vi "Decode.vi"(8 "error in (no error)":errorcluster, 10 "Clear Raw Data":bool caption="Clear Raw Data(False)", 11 "Raw Data":string) -> (0 "error out":errorcluster, 1 "Success":bool, 2 "Sequence No":string, 3 "Data":string)   [LabVIEW 2019, in "GaitDAQ UI.lvlib"]
uses:
  GaitDAQ UI.lvlib
  Step.ctl
  Sign.ctl
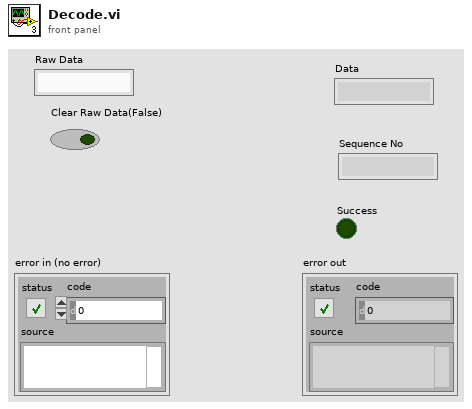
[diagram p1: front panel]
types:
  T1 = typedef "GaitDAQ UI.lvlib/Step.ctl" = enum16{"找A帧头", "找A序号", "找A数据", "找B帧头", "找B序号", "找B数据"}
  T2 = typedef "GaitDAQ UI.lvlib/Sign.ctl" = i32
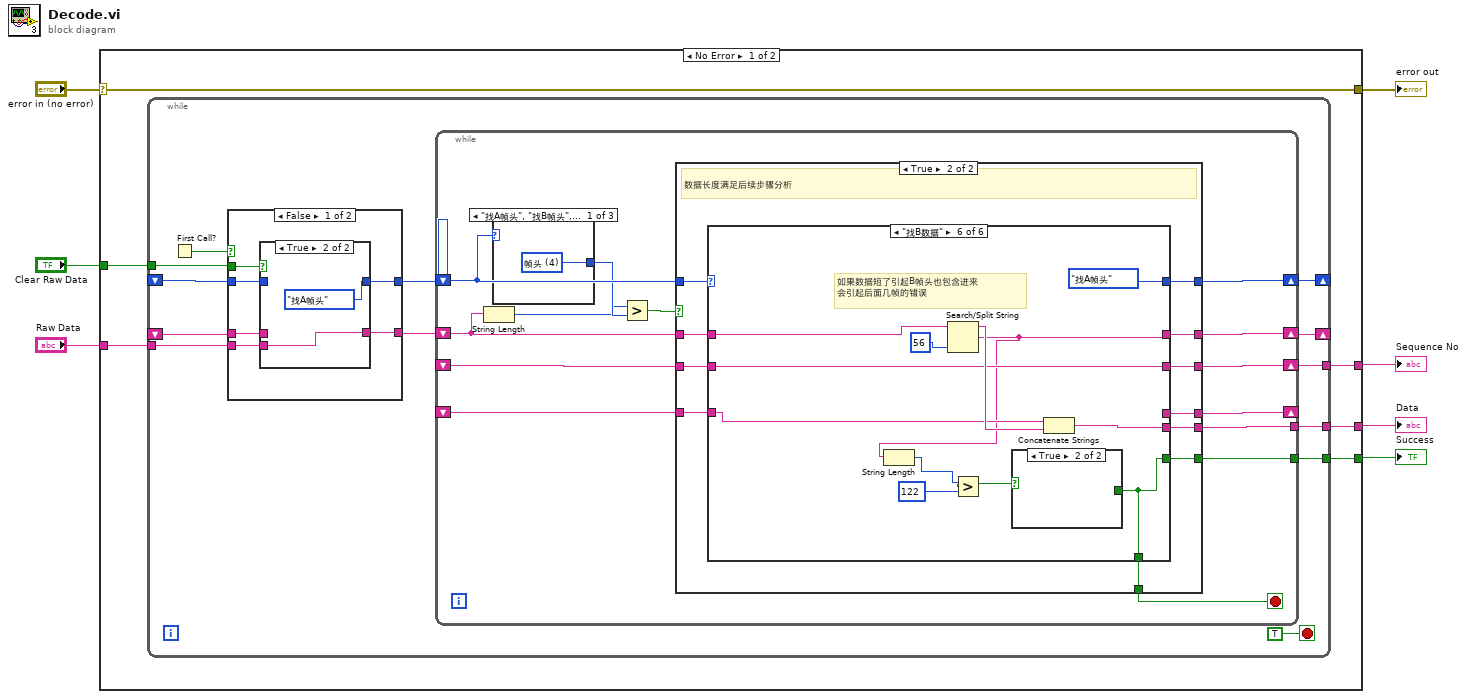
[diagram p0: block diagram]
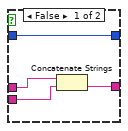
[diagram p2: hidden frame]
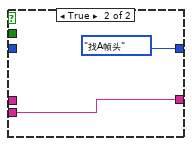
[diagram p3: hidden frame]
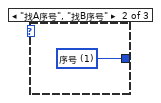
[diagram p4: hidden frame]
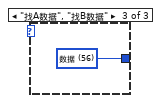
[diagram p5: hidden frame]
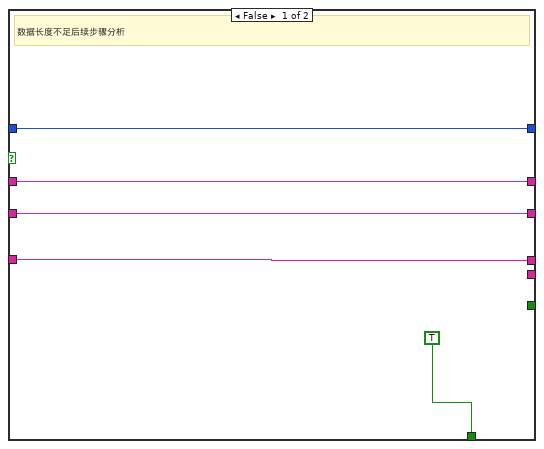
[diagram p6: hidden frame]
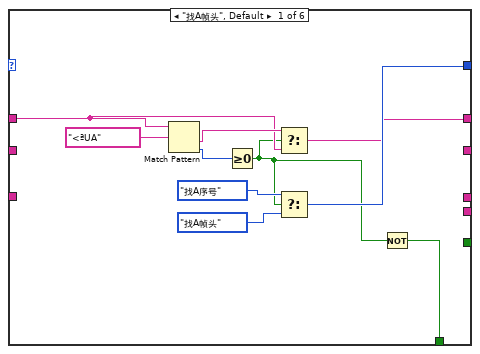
[diagram p7: hidden frame]
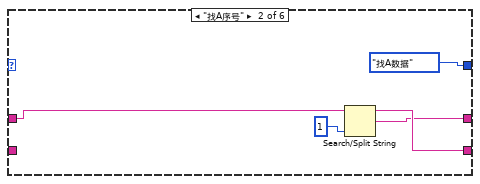
[diagram p8: hidden frame]
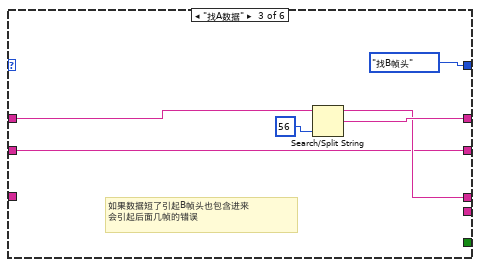
[diagram p9: hidden frame]
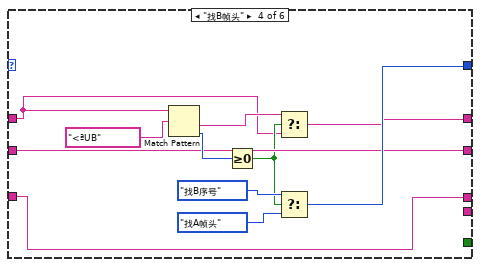
[diagram p10: hidden frame]
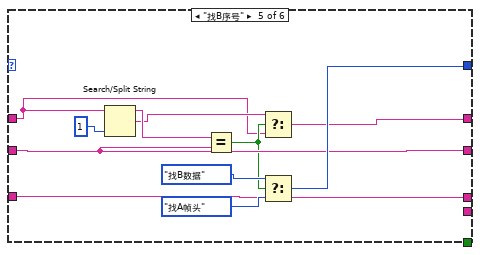
[diagram p11: hidden frame]
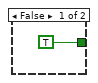
[diagram p12: hidden frame]
diagram:
  n1 = case shown="No Error" "error in (no error)" {
    selector: "error in (no error)" -> [w8 w130]
    tunnel: "Raw Data" -> [w13 _]
    tunnel: "Clear Raw Data" -> [w12 _]
    tunnel: [w11 _] -> w5
    tunnel: [w10 _] -> w4
    tunnel: [w9 _] -> w3
    tunnel: [w8 w130] -> w1
    frame No Error {
      n2 = while {
        tunnel: [w25] -> w9
        shift-right: [w26] -> _
        shift-left: _ -> [w15]
        tunnel: [w24] -> w10
        tunnel: [w23] -> w11
        tunnel: w13 -> [w16]
        tunnel: w12 -> [w17]
        shift-right: [w18] -> _
        shift-left: _ -> [w19]
        stop <- TRUE stop-if-true
        n3 = First Call?() -> (First Call?: T/F=w21:bool)
        n4 = case shown="False" w21 {
          tunnel: [w27 Step."找A帧头"] -> w20
          tunnel: w19 -> [w28 _]
          tunnel: w17 -> [w32 _]
          tunnel: w16 -> [w31 w39]
          tunnel: w15 -> [w30 _]
          tunnel: [w29 w39] -> w14
          frame False {
            n5 = case shown="True" w32 {
              tunnel: [w36 w38] -> w29
              tunnel: w31 -> [w35 w38]
              tunnel: w30 -> [w34 _]
              tunnel: w28 -> [w33 _]
              tunnel: [w33 Step."找A帧头"] -> w27
              frame False {
                n6 = Concatenate Strings(w34, w35) -> (w36:string)
              }
              frame True {
              }
            }
          }
          frame True {
          }
        }
        n7 = while {
          shift-right: [w53] -> w18
          shift-left: w20 -> [w51]
          shift-right: [w52] -> w26
          shift-left: w14 -> [w54]
          shift-right: [w46] -> w25
          shift-left: _ -> [w45]
          shift-right: [w44] -> _
          shift-left: _ -> [w43]
          tunnel: [w42] -> w23
          tunnel: [w41] -> w24
          stop <- w47 stop-if-true
          n8 = String Length(string=w54) -> (length=w49:i32)
          n9 = case shown="\"找A帧头\", \"找B帧头\", Default" w51 {
            tunnel: [w55 w56 w57] -> w50
            frame "找A帧头", "找B帧头", Default {
              w55 = T2 4 items=["帧头"=4, "序号"=1, "数据"=56]
            }
            frame "找A序号", "找B序号" {
              w56 = T2 1 items=["帧头"=4, "序号"=1, "数据"=56]
            }
            frame "找A数据", "找B数据" {
              w57 = T2 56 items=["帧头"=4, "序号"=1, "数据"=56]
            }
          }
          n10 = Greater?(x=w49, y=w50) -> (0:w48:bool)
          n11 = case shown="True" w48 {
            tunnel: w51 -> [w61 w73]
            tunnel: w54 -> [w62 w72]
            tunnel: [w61 w71] -> w53
            tunnel: [w62 w70] -> w52
            tunnel: [TRUE w67] -> w47
            tunnel: [w59 w69] -> w46
            tunnel: w45 -> [w59 w68]
            tunnel: [w58 w66] -> w44
            tunnel: w43 -> [w58 w65]
            tunnel: [_ w64] -> w42
            tunnel: [_ w63] -> w41
            frame False {
              # "数据长度不足后续步骤分析"
            }
            frame True {
              # "数据长度满足后续步骤分析"
              n12 = case shown="\"找B数据\"" w73 {
                tunnel: w72 -> [w76 w87 w90 w96 w108 w127]
                tunnel: [w80 Step."找A数据" Step."找B帧头" ("f") w102 w113 Step."找A帧头" ("f")] -> w71
                tunnel: [w78 w85 w93 w97 w107 w121] -> w70
                tunnel: [_ w86 w89 w101 w112 w122] -> w69
                tunnel: w68 -> [_ _ w89 w101 w112 w122]
                tunnel: [w75 _ _ _ _ w117] -> w67
                tunnel: [_ _ w92 w95 w106 _] -> w66
                tunnel: w65 -> [_ _ _ w95 w106 w125]
                tunnel: [_ _ _ _ _ w117] -> w64
                tunnel: [_ _ _ _ _ w123] -> w63
                frame "找A帧头", Default {
                  n13 = Match Pattern(string=w76, regular expression="<ªUA") -> (after substring=w79:string, offset past match=w82:i32)  [unwired: 1 in, 2 out]
                  n14 = Greater Or Equal To 0?(x=w82) -> (x >= 0?=w74:bool)
                  n15 = Select(t=w79, s=w74, f=w76) -> (s? t:f=w78:string)
                  n16 = Select(t=Step."找A序号", s=w74, f=Step."找A帧头") -> (s? t:f=w80:T1)
                  n17 = Not(x=w74) -> (.not. x?=w75:bool)
                }
                frame "找A序号" {
                  n18 = Search/Split String(string=w87, offset (0)=1) -> (substring before match=w86:string, match + rest of string=w85:string)  [unwired: 1 in, 1 out]
                }
                frame "找A数据" {
                  # "如果数据短了引起B帧头也包含进来\n会引起后面几帧的错误"
                  n19 = Search/Split String(string=w90, offset (0)=56) -> (substring before match=w92:string, match + rest of string=w93:string)  [unwired: 1 in, 1 out]
                }
                frame "找B帧头" {
                  n20 = Match Pattern(string=w96, regular expression="<ªUB") -> (after substring=w98:string, offset past match=w105:i32)  [unwired: 1 in, 2 out]
                  n21 = Greater Or Equal To 0?(x=w105) -> (x >= 0?=w99:bool)
                  n22 = Select(t=w98, s=w99, f=w96) -> (s? t:f=w97:string)
                  n23 = Select(t=Step."找B序号", s=w99, f=Step."找A帧头") -> (s? t:f=w102:T1)
                }
                frame "找B序号" {
                  n24 = Search/Split String(string=w108, offset (0)=1) -> (substring before match=w115:string, match + rest of string=w110:string)  [unwired: 1 in, 1 out]
                  n25 = Equal?(x=w115, y=w112) -> (x = y?=w109:bool)
                  n26 = Select(t=w110, s=w109, f=w108) -> (s? t:f=w107:string)
                  n27 = Select(t=Step."找B数据", s=w109, f=Step."找A帧头") -> (s? t:f=w113:T1)
                }
                frame "找B数据" {
                  # "如果数据短了引起B帧头也包含进来\n会引起后面几帧的错误"
                  n28 = Search/Split String(string=w127, offset (0)=56) -> (substring before match=w126:string, match + rest of string=w121:string)  [unwired: 1 in, 1 out]
                  n29 = String Length(string=w121) -> (length=w120:i32)
                  n30 = Greater?(x=w120, y=122) -> (0:w118:bool)
                  n31 = case shown="True" w118 {
                    tunnel: [TRUE _] -> w117
                    frame False {
                    }
                    frame True {
                    }
                  }
                  n32 = Concatenate Strings(w125, w126) -> (w123:string)
                }
              }
            }
          }
        }
      }
    }
    frame Error {
    }
  }
  "error out" <- w1
  "Sequence No" <- w3
  "Data" <- w4
  "Success" <- w5
